vi "PusherRefSelector.vi"(10 "PusherRefs":T1) -> (2 "Refnum":string)   [LabVIEW 2014, in "PusherLib.lvlib"]
uses:
  PusherLib.lvlib
  PusherRefs.ctl
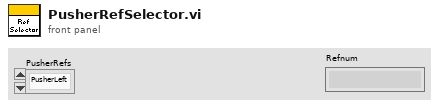
[diagram p1: front panel]
types:
  T1 = typedef "PusherLib.lvlib/PusherRefs.ctl" = enum16{"PusherLeft", "PusherRight"}
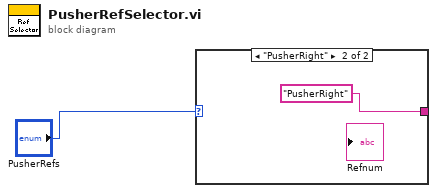
[diagram p0: block diagram]
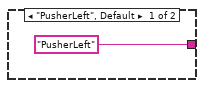
[diagram p2: hidden frame]
diagram:
  n1 = case shown="\"PusherRight\"" "PusherRefs" {
    tunnel: ["PusherLeft" "PusherRight"] -> _
    frame "PusherLeft", Default {
    }
    frame "PusherRight" {
    }
  }
